vi "CTRE_PigeonIMU_GetFusedHeading.vi"(8 "error in (no error)":errorcluster, 11 "PigeonIMUDevRef":T1={"DeviceStatus"={"status"=FALSE, "code"=0, "source"=""}, "Device Number"=0, "Type"=352321536, "Device ID"=0, "Handle"=0, "UsageFrame"=0, "Library Path"=path ""} {"Type" items=["CAN"=352321536, "TalonSRX"=33554432]}) -> (0 "error out":errorcluster, 2 "Fused Heading":T3, 3 "PigeonIMUDevRef":T1={"DeviceStatus"={"status"=FALSE, "code"=0, "source"=""}, "Device Number"=0, "Type"=352321536, "Device ID"=0, "Handle"=0, "UsageFrame"=0, "Library Path"=path ""} {"Type" items=["CAN"=352321536, "TalonSRX"=33554432]})   [LabVIEW 2016]
uses:
  <vilib>/Rock Robotics/WPI/ThirdParty/Sensors/Pigeon IMU/CTRE_PigeonIMU_DeviceRef.ctl
  <vilib>/Rock Robotics/WPI/ThirdParty/Sensors/Pigeon IMU/CTRE_PigeonIMU_ConnectionType.ctl
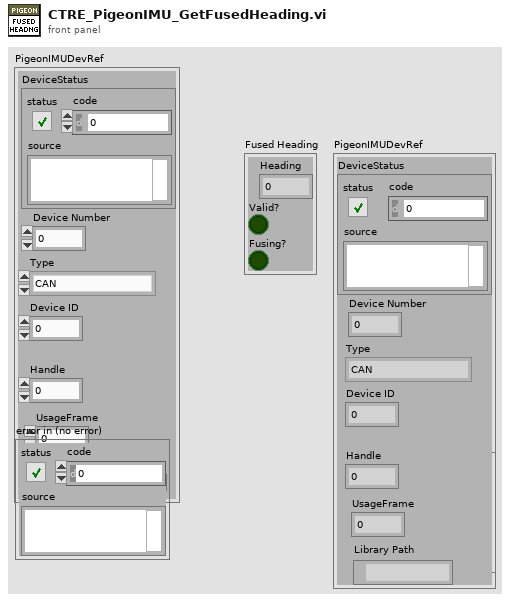
[diagram p1: front panel]
types:
  T1 = typedef "CTRE_PigeonIMU_DeviceRef.ctl" = cluster{"DeviceStatus":errorcluster, "Device Number":u8, "Type":T2, "Device ID":u32, "Handle":u64, "UsageFrame":u32, "Library Path":path}
  T2 = typedef "CTRE_PigeonIMU_ConnectionType.ctl" = u32
  T3 = cluster{"Heading":dbl, "Valid?":bool, "Fusing?":bool}
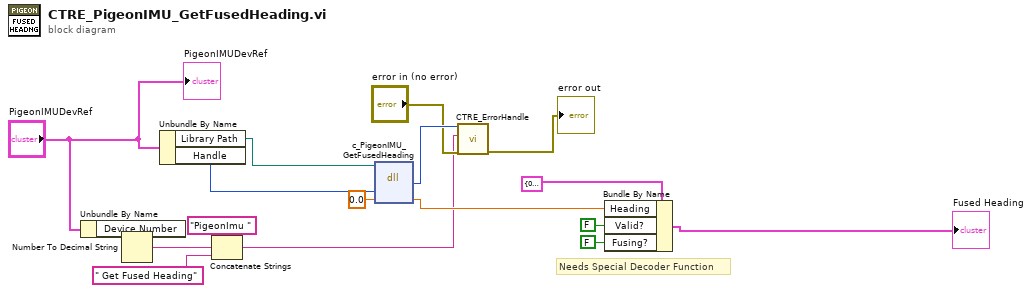
[diagram p0: block diagram]
diagram:
  # "Needs Special Decoder Function"
  n1 = Unbundle By Name("PigeonIMUDevRef") -> ("Device Number"=w6:u8)
  n2 = Number To Decimal String(number=w6) -> (decimal integer string=w5:string)  [unwired: 1 in]
  n3 = Unbundle By Name("PigeonIMUDevRef") -> ("Library Path"=w15:path, "Handle"=w14:u64)
  n4 = Concatenate Strings("PigeonImu " ("string"), w5, " Get Fused Heading" ("string")) -> (w2:string)
  n5 = dll-call lib="?" fn="c_PigeonIMU_GetFusedHeading"(path in=w15, "handle"=w14, "value"=0.0) -> ("return type"=w9:i32, "value"=w16:dbl)  [unwired: 3 in, 2 out]
  n6 = call <vilib>:"CTRE_ErrorHandle.vi"("error in"="error in (no error)", "origin"=w2, "code"=w9) -> ("error out"=→"error out":errorcluster)  [unwired: 8 in]
  n7 = Bundle By Name(cluster=T3 {"Heading"=0.0, "Valid?"=FALSE, "Fusing?"=FALSE} ("FusedHeading"), "Heading"=w16, "Valid?"=FALSE, "Fusing?"=FALSE) -> (→"Fused Heading":T3)
  "PigeonIMUDevRef" <- "PigeonIMUDevRef"
